vi "Hide Wifi Networks.vi"() -> ()   [LabVIEW 2024]
uses:
  Controls/Network.ctl
panel:
  in  "Toggle":bool
  out "Results":string[](array[string])
  in  "Submit":bool
  in  "SSID Values":T1[](array[typedef])=[{"SSID"="Network", "Pswd?"=FALSE, "Hide?"=FALSE}, {"SSID"="MONU_SIGN_HUB", "Pswd?"=FALSE, "Hide?"=FALSE}, {"SSID"="UHS-GUEST", "Pswd?"=FALSE, "Hide?"=FALSE}, {"SSID"="UHS", "Pswd?"=FALSE, "Hide?"=FALSE}, {"SSID"="MB", "Pswd?"=FALSE, "Hide?"=FALSE}, {"SSID"="MYCAR6741", "Pswd?"=FALSE, "Hide?"=FALSE}, {"SSID"="Justinƒ?Ts", "Pswd?"=FALSE, "Hide?"=FALSE}, {"SSID"="InDemand", "Pswd?"=TRUE, "Hide?"=FALSE}, {"SSID"="RTC-Transit-VLAN", "Pswd?"=FALSE, "Hide?"=FALSE}]
  out "standard output":string
  # "Notes:\n1. Open settings and scan wifi to display full set\n2. Run as admin"
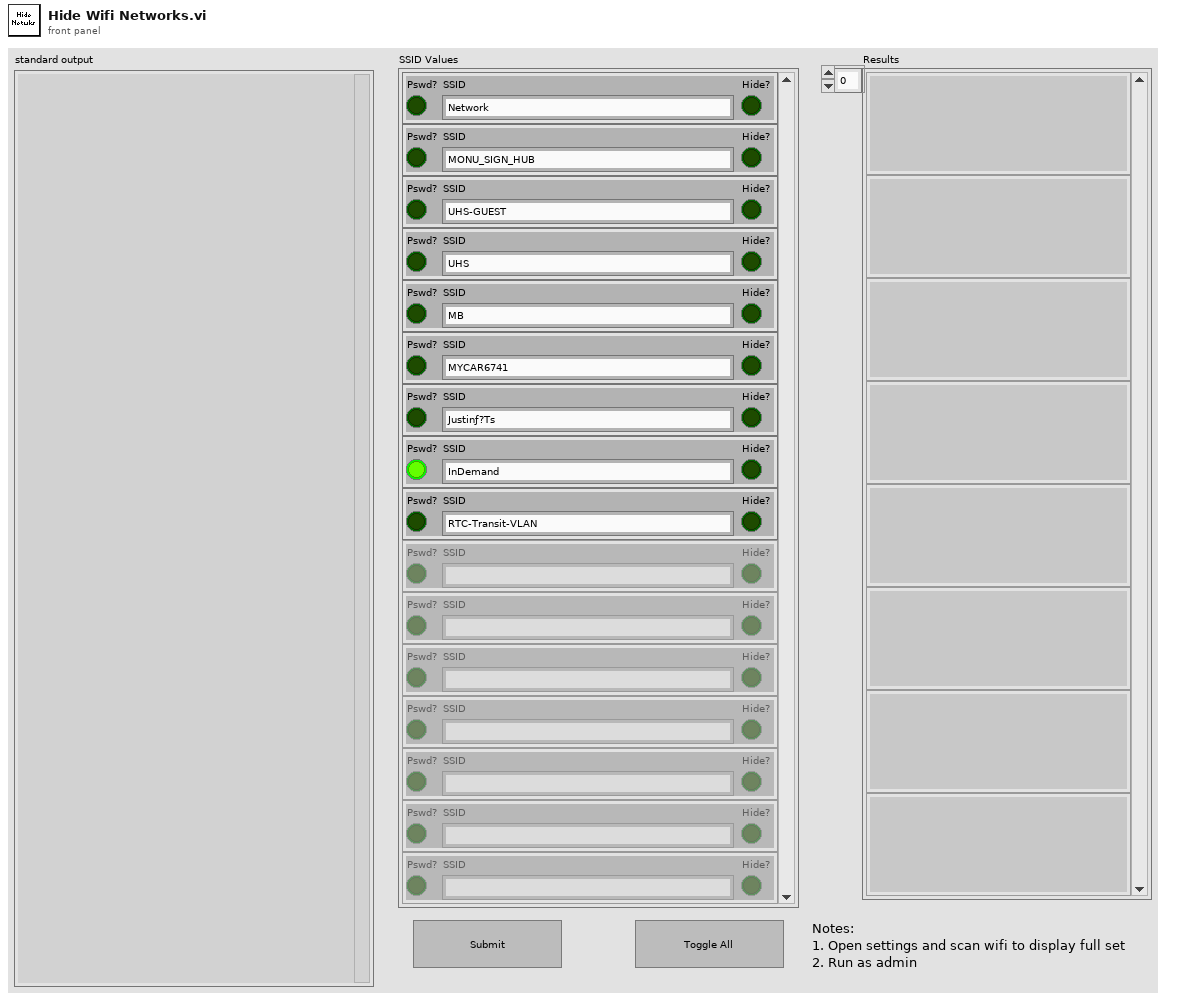
[diagram p1: front panel]
types:
  T1 = typedef "Network.ctl" = cluster{"SSID":string, "Pswd?":bool, "Hide?":bool}
  T2 = enum8{"Enabled", "Disabled", "Disabled and Grayed Out"}
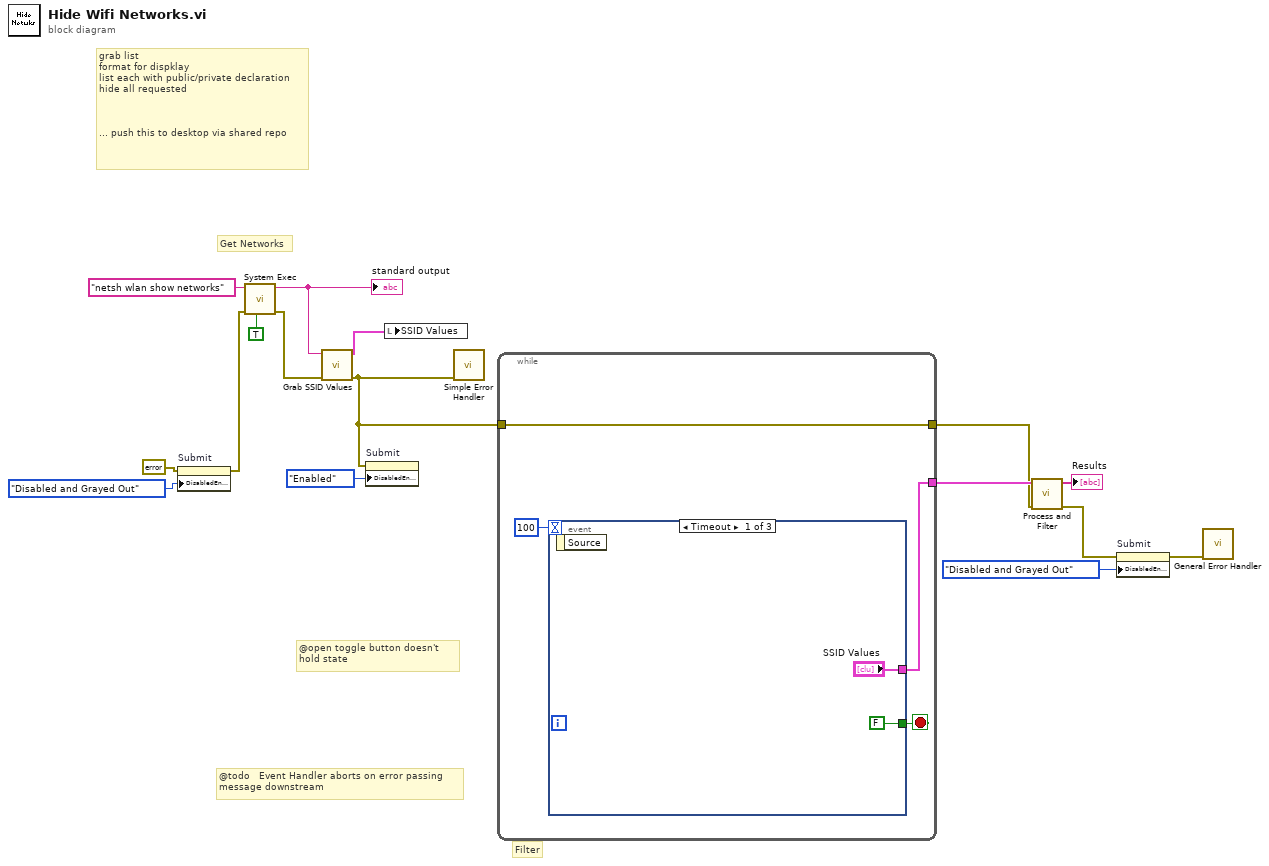
[diagram p0: block diagram]
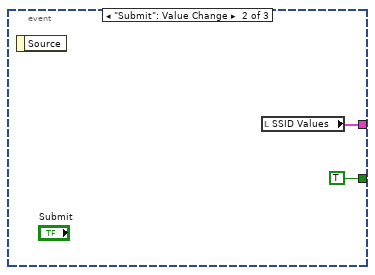
[diagram p2: hidden frame]
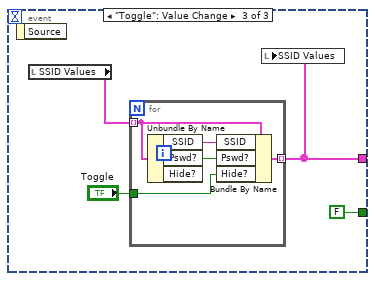
[diagram p3: hidden frame]
diagram:
  # "@open toggle button doesn't \nhold state"
  # "@todo   Event Handler aborts on error passing\nmessage downstream"
  # "Filter"
  # "Get Networks"
  # "grab list\nformat for dispklay\nlist each with public/private declaration\nhide all requested\n\n\n\n... push this to desktop via shared repo"
  n1 = property on="Submit" class="Bool"(error in=errorcluster {"status"=FALSE, "code"=0, "source"=""} ("error in (no error)"), "DisabledEnum"=T2."Disabled and Grayed Out" ("Disabled")) -> (error out=w9:errorcluster)  [unwired: 1 in, 1 out]
  n2 = call <vilib>:"System Exec.vi"("run minimized? (F)"=TRUE, "error in (no error)"=w9, "command line"="netsh wlan show networks") -> ("error out"=w14:errorcluster, "standard output"=w15:string)  [unwired: 5 in, 2 out]
  "standard output" <- w15
  n3 = call "Grab SSID Values.vi"("error in (no error)"=w14, "standard output"=w15) -> ("error out"=w8:errorcluster, "SSID Values"=w1:T1[])  [unwired: 7 in, 1 out]
  n4 = property on="Submit" class="Bool"(error in=w8, "DisabledEnum"=T2."Enabled" ("Disabled")) -> ()  [unwired: 1 in, 2 out]
  n5 = local write "SSID Values"(w1) -> ()
  n6 = call <vilib>:"Simple Error Handler.vi"("error in (no error)"=w8) -> ()  [unwired: 4 in, 5 out]
  n7 = while {
    tunnel: w8 -> [w20]
    tunnel: [w20] -> w5
    tunnel: [w17] -> w6
    stop <- w19 stop-if-true
    n8 = event shown="[0] Timeout" {
      selector: _ -> [_ _ _]
      dyn-events: _ -> [_ _ _]
      timeout: u32 100 ("milliseconds to wait") -> [_ _ _]
      tunnel: [FALSE TRUE FALSE] -> w19
      tunnel: ["SSID Values" w23 w26] -> w17
      event Timeout {
        n9 = event-data() -> ()  [unwired: 1 in, 1 out]
      }
      event "Submit": Value Change {
        n10 = event-data() -> ()  [unwired: 1 in, 1 out]
        n11 = local read "SSID Values"() -> (w23:T1[])
      }
      event "Toggle": Value Change {
        n12 = event-data() -> ()  [unwired: 1 in, 1 out]
        n13 = local read "SSID Values"() -> (w28:T1[])
        n14 = for {
          tunnel: w28 -> [w33] mode=indexing
          tunnel: [w30] -> w26 mode=indexing
          tunnel: "Toggle" -> [w29]
          n15 = Unbundle By Name(w33) -> ("SSID"=w32:string, "Pswd?"=w31:bool)  [unwired: 1 out]
          n16 = Bundle By Name(cluster=w33, "SSID"=w32, "Pswd?"=w31, "Hide?"=w29) -> (w30:T1)
        }
        n17 = local write "SSID Values"(w26) -> ()
      }
    }
  }
  n18 = call "Process and Filter.vi"("error in (no error)"=w5, "SSID Values"=w6) -> ("error out"=w4:errorcluster, "Results"=→"Results":string[])  [unwired: 8 in]
  n19 = property on="Submit" class="Bool"(error in=w4, "DisabledEnum"=T2."Disabled and Grayed Out" ("Disabled")) -> (error out=w3:errorcluster)  [unwired: 1 in, 1 out]
  n20 = call <vilib>:"General Error Handler.vi"("error in (no error)"=w3) -> ()  [unwired: 10 in, 5 out]
